vi "Dispose DataColumns.vi"(8 "error in (no error)":errorcluster caption="错误输入（无错误）", 11 "DataColumns":refnum<class "Data Column.lvclass">[](array[class])) -> (0 "error out":errorcluster caption="错误输出")   [LabVIEW 2012, in "Data Grid VIEW.lvlib" / "Data Column.lvclass"]
uses:
  Data Column.lvclass
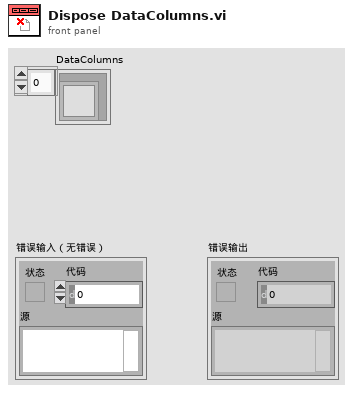
[diagram p1: front panel]
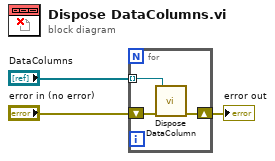
[diagram p0: block diagram]
diagram:
  n1 = for {
    tunnel: "DataColumns" -> [w6] mode=indexing
    shift-right: [w4] -> w1
    shift-left: "error in (no error)" -> [w5]
    n2 = call "Dispose DataColumn.vi"("error in (no error)"=w5, "Data Column 输入"=w6) -> ("error out"=w4:errorcluster)  [unwired: 8 in, 1 out]
  }
  "error out" <- w1
